vi "RM.applyWindowSettings.vi"(8 "error in (no error)":errorcluster, 11 "VI reference":refnum<vi>) -> (0 "error out":errorcluster)   [LabVIEW 2016, in "FPGA Resource Manager.lvlib"]
uses:
  FPGA Resource Manager.lvlib
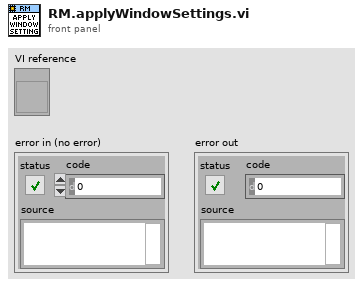
[diagram p1: front panel]
types:
  T1 = enum32{"Invalid", "Standard", "Closed", "Hidden", "Minimized", "Maximized"}
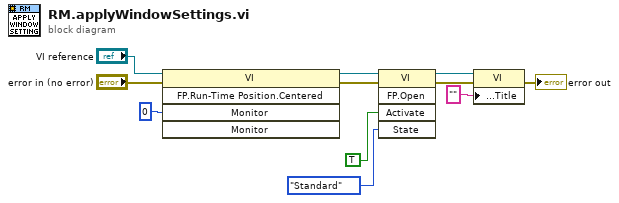
[diagram p0: block diagram]
diagram:
  n1 = invoke class="VI" method="FP.Run-Time Position.Centered"(reference="VI reference", error in="error in (no error)", "Monitor"=i16 0) -> (reference out=w5:refnum<vi>, error out=w4:errorcluster)  [unwired: 2 in, 3 out]
  n2 = invoke class="VI" method="FP.Open"(reference=w5, error in=w4, "Activate"=TRUE ("Activate?"), "State"=T1."Standard") -> (reference out=w10:refnum<vi>, error out=w8:errorcluster)  [unwired: 1 in, 3 out]
  n3 = property class="VI"(reference=w10, error in=w8, "Front Panel.Title"="" ("Front Panel Window:Title")) -> (error out=→"error out":errorcluster)  [unwired: 1 out]
